vi "Initialize.vi"(6 "Actor Name":string, 7 "Host Name":string, 8 "error in (no error)":errorcluster, 10 "Application Data":path, 11 "Message Broker":refnum<class "Message Broker Interface Ref.lvclass">) -> (0 "error out":errorcluster, 3 "Bank Account out":refnum<class "Bank Account.lvclass">)   [LabVIEW 2016, in "CLD Exam - ATM.lvlib" / "Bank Account.lvclass"]
uses:
  Bank Account.lvclass
  Mediator/Classes/Message Broker Interface Ref/Message Broker Interface Ref.lvclass
  D:/Repos/Stream/software/Mediator/Classes/Message Broker Interface/Message Broker Interface.lvclass
  Bank Account.lvclass/Bank Account.ctl
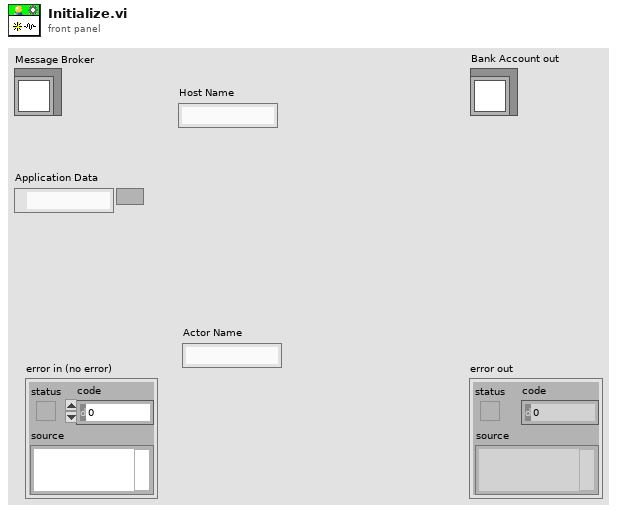
[diagram p1: front panel]
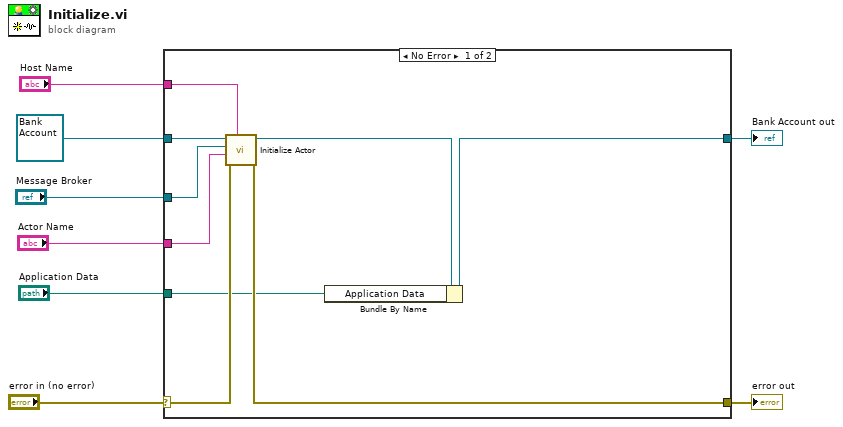
[diagram p0: block diagram]
diagram:
  n1 = case shown="No Error" "error in (no error)" {
    selector: "error in (no error)" -> [w16 w19]
    tunnel: [w15 w19] -> w7
    tunnel: [w9 w18] -> w5
    tunnel: refnum<class "Bank Account.lvclass"> refnum ("Bank Account in") -> [w17 w18]
    tunnel: "Host Name" -> [w14 _]
    tunnel: "Message Broker" -> [w13 _]
    tunnel: "Actor Name" -> [w12 _]
    tunnel: "Application Data" -> [w11 _]
    frame No Error {
      n2 = call-dynamic "Initialize Actor.vi"("Host Name"=w14, "error in (no error)"=w16, "Actor Name"=w12, "Message Broker Interface"=w13, "Bank Account in"=w17) -> ("error out"=w15:errorcluster, "Bank Account out"=w10:refnum<class "Bank Account.lvclass">)  [unwired: 5 in]
      n3 = Bundle By Name(cluster=w10, "Application Data"=w11) -> (w9:refnum<class "Bank Account.lvclass">)
    }
    frame Error {
    }
  }
  "error out" <- w7
  "Bank Account out" <- w5
